vi "GFITS_Parse Arithmetic Expression.vi"(3 "Arithmetic Expression":string="1 + 3.1415 * 2*2") -> (0 "Result":dbl format="%.6f", 1 "string_result":string)   [LabVIEW 2016]
doc: "This somewhat more advanced example VI shows how to use the Scan String for Tokens and Scan From String primitives to write an infix arithmetic expression parser."
panel:
  # "Arithmetic expression (infix) parser"
  # "Enter an arithmetic expression into the control below.  Known operators are: +, -, *, /, %, (, )\nPress <ctrl-h> for more information."
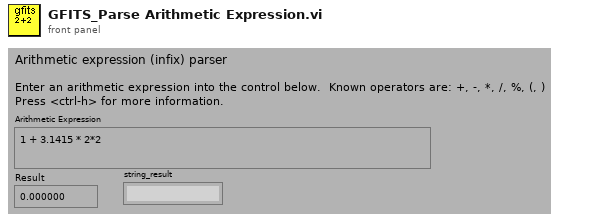
[diagram p1: front panel]
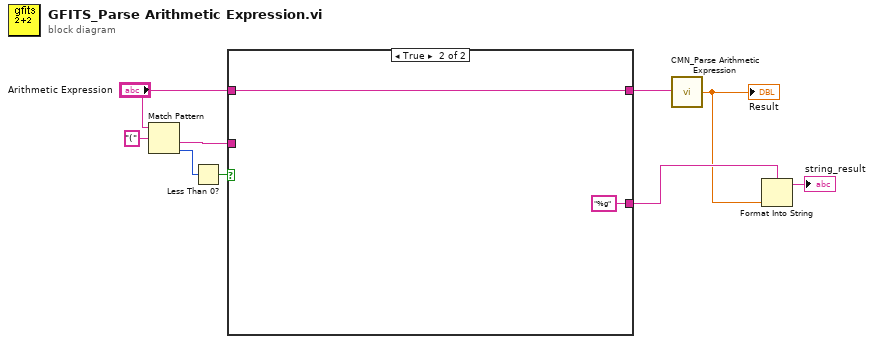
[diagram p0: block diagram]
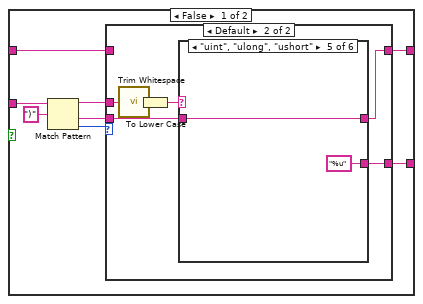
[diagram p2: hidden frame]
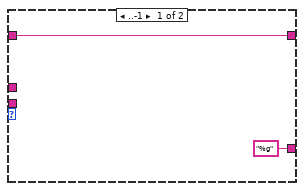
[diagram p3: hidden frame]
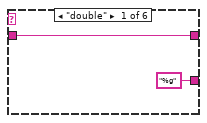
[diagram p4: hidden frame]
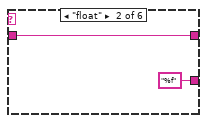
[diagram p5: hidden frame]
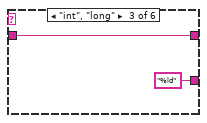
[diagram p6: hidden frame]
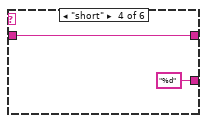
[diagram p7: hidden frame]
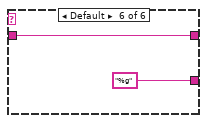
[diagram p8: hidden frame]
diagram:
  n1 = Match Pattern(string="Arithmetic Expression", regular expression="(") -> (after substring=w8:string, offset past match=w2:i32)  [unwired: 3 out]
  n2 = Less Than 0?(x=w2) -> (x < 0?=w1:bool)
  n3 = case shown="True" w1 {
    tunnel: w8 -> [w17 _]
    tunnel: "Arithmetic Expression" -> [w14 w39]
    tunnel: [w13 w39] -> w6
    tunnel: [w10 "%g" ("Arithmetic Expression")] -> w5
    frame False {
      n4 = Match Pattern(string=w17, regular expression=")") -> (before substring=w12:string, after substring=w11:string, offset past match=w15:i32)  [unwired: 2 out]
      n5 = case shown="Default" w15 {
        tunnel: w14 -> [w19 _]
        tunnel: [w19 w20] -> w13
        tunnel: w12 -> [_ w25]
        tunnel: w11 -> [_ w21]
        tunnel: ["%g" ("Arithmetic Expression") w22] -> w10
        frame ..-1 {
        }
        frame Default {
          n6 = call <vilib>:"Trim Whitespace.vi"("string"=w25) -> ("trimmed string"=w24:string)  [unwired: 1 in]
          n7 = To Lower Case(string=w24) -> (all lower case string=w23:string)
          n8 = case shown="\"uint\", \"ulong\", \"ushort\"" w23 {
            tunnel: ["%g" ("Arithmetic Expression") "%f" ("Arithmetic Expression") "%ld" ("Arithmetic Expression") "%d" ("Arithmetic Expression") "%u" ("Arithmetic Expression") "%g" ("Arithmetic Expression")] -> w22
            tunnel: w21 -> [w27 w29 w31 w33 w35 w36]
            tunnel: [w27 w29 w31 w33 w35 w36] -> w20
            frame "double" {
            }
            frame "float" {
            }
            frame "int", "long" {
            }
            frame "short" {
            }
            frame "uint", "ulong", "ushort" {
            }
            frame Default {
            }
          }
        }
      }
    }
    frame True {
    }
  }
  n9 = call "CMN_Parse Arithmetic Expression.vi"("Arithmetic Expression"=w6) -> ("Result"=w4:dbl)
  "Result" <- w4
  n10 = Format Into String(format string=w5, w4) -> (resulting string=→"string_result":string)  [unwired: 2 in, 1 out]
